vi "Step Update Table 4.0 to 4.1.vi"(8 "error in (no error)":errorcluster, 11 "Connection Refnum":T1) -> (0 "error out":errorcluster, 3 "Connection Refnum Out":T1)   [LabVIEW 2011]
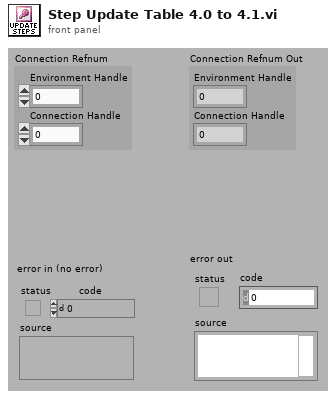
[diagram p1: front panel]
types:
  T1 = cluster{"Environment Handle":i32, "Connection Handle":i32}
  T2 = typedef "Statement Refnum.ctl" = cluster{"Statement Handle":i32, "Parameter Number":u16}
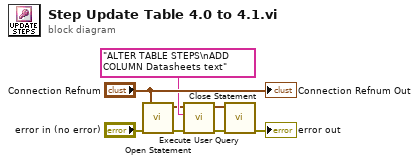
[diagram p0: block diagram]
diagram:
  n1 = call "Open Statement.vi"("error in (no error)"="error in (no error)", "Connection Refnum"="Connection Refnum") -> ("error out"=w1:errorcluster, "Statement Refnum"=w2:T2)  [unwired: 4 out]
  n2 = call "Execute User Query.vi"("error in (no error)"=w1, "User Query"="ALTER TABLE STEPS\nADD COLUMN Datasheets text", "Statement Refnum"=w2) -> ("error out"=w4:errorcluster, "Statement Refnum"=w5:T2)  [unwired: 1 in, 2 out]
  n3 = call "Close Statement.vi"("error in (no error)"=w4, "Statement Refnum"=w5) -> ("error out"=→"error out":errorcluster)  [unwired: 5 out]
  "Connection Refnum Out" <- "Connection Refnum"
